vi "initObjectArray.vi"() -> (3 "CheckData out":refnum<class "CheckData.lvclass">[](array[class]))   [LabVIEW 2017, in "CheckData.lvclass"]
uses:
  CheckData.lvclass
  DAQ/Master_DataControl.ctl
  DAQ/TypeDef_cRIOData.ctl
  IMU/TypeDef_IMUData.ctl
  CAN/TypeDef_BMSData.ctl
  CAN/TypeDef_BMS_Status.ctl
  CAN/MotorController/fixedMotorData.ctl
  CAN/MotorController/MotorStatus.ctl
  CheckData.lvclass/CheckData.ctl
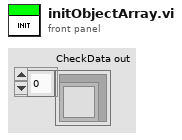
[diagram p1: front panel]
types:
  T1 = typedef "Master_DataControl.ctl" = cluster{"cRIO Data":T2, "IMU Data":T3, "BMS Data":T4, "Motor Data":T6}
  T2 = typedef "TypeDef_cRIOData.ctl" = cluster{"Time (ms)":dbl, "24V Battery (V)":dbl, "LowV Current (A)":dbl, "Fiducial Sensor (V)":dbl, "PV Pressure (psig)":dbl, "Flow Sensor (V)":dbl, "Temp Fairing (F)":dbl, "Temp Reservoir (F)":dbl, "HallEffect Right (in)":dbl, "HallEffect Left (in)":dbl, "PT Tank (psig)":dbl, "PT Clamp Right (psig)":dbl, "PT Clamp Left (psig)":dbl, "PT Brake (psig)":dbl, "PT Cooling (psig)":dbl, "Displacement (ft)":dbl, "Velocity (ft/s)":dbl}
  T3 = typedef "TypeDef_IMUData.ctl" = cluster{"x acceleration (g)":dbl, "Pressure (psia)":dbl, "Temperature (F)":dbl}
  T4 = typedef "TypeDef_BMSData.ctl" = cluster{"Max Cell Voltage (V)":dbl, "Max Cell ID":dbl, "Min Cell Voltage (V)":dbl, "Min Cell ID":dbl, "State of Charge (%)":dbl, "Average Voltage (V)":dbl, "Voltage Delta (V)":dbl, "Pack Current (A)":dbl, "Pack Voltage (V)":dbl, "Max Resistance (Ohm)":dbl, "Min Resistance (Ohm)":dbl, "Average Resistance (Ohm)":dbl, "Delta Resistance (Ohm)":dbl, "Highest Temperature(F)":dbl, "BmsStatus":T5}
  T5 = typedef "TypeDef_BMS_Status.ctl" = cluster{"isFault":bool, "isolationMonitoring":bool}
  T6 = typedef "fixedMotorData.ctl" = cluster{"Velo (RPM)":dbl, "MotorTemp(F)":dbl, "CtrlTemp(F)":dbl, "DcLinkVolt(V)":dbl, "ErrorCode":dbl, "motorStatus":T7, "isAlive":bool, "motorControllerState":u16}
  T7 = typedef "MotorStatus.ctl" = cluster{"isReady":bool, "isOn":bool, "isOperEn":bool, "isFault":bool, "isVoltEn":bool, "targetReached":bool, "isWarning":bool}
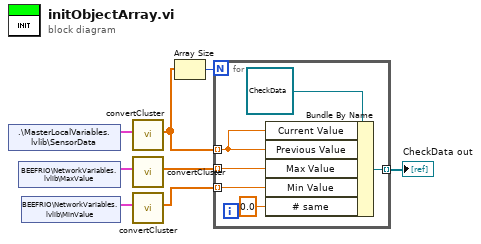
[diagram p0: block diagram]
diagram:
  n1 = shared-variable ".\\MasterLocalVariables.lvlib\\SensorData"() -> (w2:T1)  [unwired: 1 in, 1 out]
  n2 = shared-variable "BEEFRIO\\NetworkVariables.lvlib\\MaxValue"() -> (w7:T1)  [unwired: 1 in, 1 out]
  n3 = shared-variable "BEEFRIO\\NetworkVariables.lvlib\\MinValue"() -> (w6:T1)  [unwired: 1 in, 1 out]
  n4 = call "convertCluster.vi"("Data"=w2) -> ("Array"=w1:dbl[])  [unwired: 10 in]
  n5 = call "convertCluster.vi"("Data"=w7) -> ("Array"=w5:dbl[])  [unwired: 10 in]
  n6 = call "convertCluster.vi"("Data"=w6) -> ("Array"=w4:dbl[])  [unwired: 10 in]
  n7 = Array Size(array=w1) -> (size(s)=w8:i32)
  n8 = for {
    N: w8 -> [_]
    tunnel: w1 -> [w13] mode=indexing
    tunnel: w5 -> [w12] mode=indexing
    tunnel: w4 -> [w11] mode=indexing
    tunnel: [w10] -> w3 mode=indexing
    n9 = Bundle By Name(cluster=refnum<class "CheckData.lvclass"> refnum ("CheckData out"), "Current Value"=w13, "Previous Value"=w13, "Max Value"=w12, "Min Value"=w11, "# same"=0.0) -> (w10:refnum<class "CheckData.lvclass">)
  }
  "CheckData out" <- w3
